vi "Get By Challenge and User.vi"(8 "error in (no error)":errorcluster, 9 "Challenge ID":i64, 10 "User ID":i64, 11 "Submission DB in":refnum<class "Submission DB.lvclass">) -> (0 "error out":errorcluster, 2 "Submissions":refnum<class "Submission.lvclass">[](array[class]), 3 "Submission DB out":refnum<class "Submission DB.lvclass">)   [LabVIEW 2020, in "Summer of LabVIEW.lvlib" / "Submission DB.lvclass"]
uses:
  Submission DB.lvclass
  Submission/Submission.lvclass
  Submission DB.lvclass/Submission DB.ctl
  <vilib>/drjdpowell/SQLite Library/SQL Statement/SQL Statement.lvclass/SQL Statement.ctl
  <vilib>/drjdpowell/SQLite Library/SQL Statement/Bind Integer.vi
  <vilib>/drjdpowell/SQLite Library/SQL Statement/Finalize.vi
  <vilib>/drjdpowell/SQLite Library/SQL Statement/Error Message.vi
  <vilib>/drjdpowell/SQLite Library/SQL Statement/SQL Statement.lvclass
  SQLite/SQLite.lvclass
  <vilib>/drjdpowell/SQLite Library/SQL Connection/Connection.lvclass
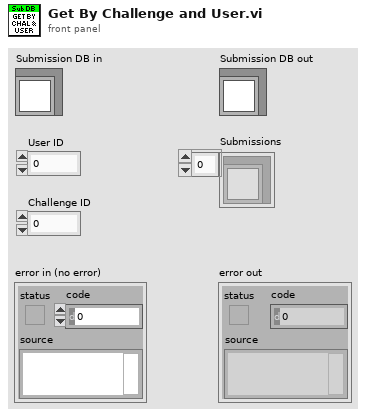
[diagram p1: front panel]
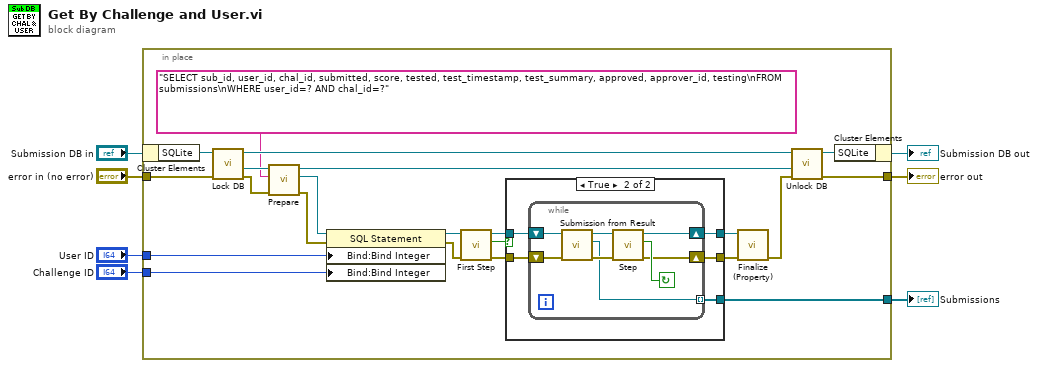
[diagram p0: block diagram]
diagram:
  n1 = in-place {
    in-place-border: "error in (no error)" -> [w27]
    in-place-border: [w24] -> w5
    in-place-border: [w18] -> w3
    in-place-border: "User ID" -> [w13]
    in-place-border: "Challenge ID" -> [w12]
    n2 = in-place-cluster #1("Submission DB in") -> ("SQLite"=w28:refnum<class "SQLite.lvclass">)
    n3 = call "Lock DB.vi"("error in (no error)"=w27, "SQLite in"=w28) -> ("error out"=w29:errorcluster, "SQLite DB"=w23:refnum<class "Connection.lvclass">, "SQLite out"=w25:refnum<class "SQLite.lvclass">)  [unwired: 6 in, 1 out]
    n4 = call <vilib>:"Prepare.vi"("error in (no error)"=w29, "SQL"="SELECT sub_id, user_id, chal_id, submitted, score, tested, test_timestamp, test_summary, approved, approver_id, testing\nFROM submissions\nWHERE user_id=? AND chal_id=?", "SQLite Connection in"=w23) -> ("error out"=w14:errorcluster, "SQL Statement"=w17:refnum<class "SQL Statement.lvclass">, "SQLite Connection"=w8:refnum<class "Connection.lvclass">)  [unwired: 4 in, 2 out]
    n5 = property class="SQL Statement"(reference=w17, error in=w14, "Bind:Bind Integer"=w13, "Bind:Bind Integer"=w12) -> (reference out=w16:refnum<class "SQL Statement.lvclass">, error out=w15:errorcluster)
    n6 = call <vilib>:"First Step.vi"("error in (no error)"=w15, "SQL Statement in"=w16) -> ("error out"=w19:errorcluster, "Row returned"=w21:bool, "SQL Statement"=w20:refnum<class "SQL Statement.lvclass">)  [unwired: 7 in]
    n7 = case shown="True" w21 {
      tunnel: w20 -> [w31 w36]
      tunnel: w19 -> [w30 w35]
      tunnel: [_ w34] -> w18
      tunnel: [w31 w33] -> w11
      tunnel: [w30 w32] -> w10
      frame False {
      }
      frame True {
        n8 = while {
          shift-right: [w42] -> w33
          shift-left: w36 -> [w41]
          shift-right: [w43] -> w32
          shift-left: w35 -> [w40]
          tunnel: [w37] -> w34 mode=indexing
          stop <- w44 continue-if-true
          n9 = call "Submission from Result.vi"("error in (no error)"=w40, "Statement In"=w41) -> ("error out"=w38:errorcluster, "Submission"=w37:refnum<class "Submission.lvclass">, "Statement"=w39:refnum<class "SQL Statement.lvclass">)  [unwired: 7 in]
          n10 = call <vilib>:"Step.vi"("error in (no error)"=w38, "SQL Statement in"=w39) -> ("error out"=w43:errorcluster, "Row returned"=w44:bool, "SQL Statement"=w42:refnum<class "SQL Statement.lvclass">)  [unwired: 7 in]
        }
      }
    }
    n11 = call <vilib>:"Finalize (Property).vi"("error in (no error)"=w10, "SQL Statement in"=w11) -> ("error out"=w9:errorcluster)  [unwired: 7 in, 2 out]
    n12 = call "Unlock DB.vi"("error in (no error)"=w9, "SQLite DB"=w8, "SQLite in"=w25) -> ("error out"=w24:errorcluster, "SQLite out"=w26:refnum<class "SQLite.lvclass">)  [unwired: 7 in]
    n13 = in-place-cluster #1("SQLite"=w26) -> (→"Submission DB out":refnum<class "Submission DB.lvclass">)
  }
  "error out" <- w5
  "Submissions" <- w3
